vi "Message type.vi"(11 "MsgPackMessage in":refnum<class "WampMessage MsgPack.lvclass">) -> (2 "Message Codes":T1, 3 "MsgPackMessage out":refnum<class "WampMessage MsgPack.lvclass">)   [LabVIEW 2020, in "wamplv.lvlib" / "WampMessage MsgPack.lvclass"]
uses:
  WampMessage MsgPack.lvclass
  TypeDefs/WAMP Message Codes.ctl
  WampMessage MsgPack.lvclass/WampMessage MsgPack.ctl
  wamplv.lvlib
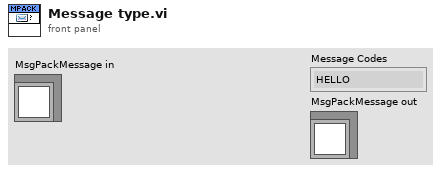
[diagram p1: front panel]
types:
  T1 = typedef "wamplv.lvlib/WAMP Message Codes.ctl" = enum8{"HELLO", "WELCOME", "CHALLENGE", "AUTHENTICATE", "ABORT", "GOODBYE", "ERROR", "PUBLISH", "PUBLISHED", "SUBSCRIBE", "SUBSCRIBED", "UNSUBSCRIBE", "UNSUBSCRIBED", "EVENT", "CALL", "RESULT", "REGISTER", "REGISTERED", "UNREGISTER", "UNREGISTERED", "INVOCATION", "YIELD"}
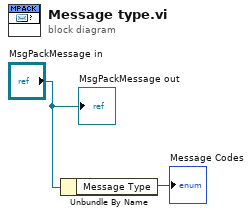
[diagram p0: block diagram]
diagram:
  n1 = Unbundle By Name("MsgPackMessage in") -> ("Message Type"=→"Message Codes":T1)
  "MsgPackMessage out" <- "MsgPackMessage in"
